vi "SaveAs Document.vi"(8 "error in (no error)":errorcluster, 10 "File Path":path, 11 "Document in":refnum<class "Document.lvclass">) -> (0 "error out":errorcluster, 3 "Document out":refnum<class "Document.lvclass">)   [LabVIEW 2020, in "LabVIEW NPOI.lvlib" / "Document.lvclass"]
doc: "Saves the <b>Document</b> to the given <b>File Path</b>.\n\nNotes:\n - If <b>File Path</b> is empty (default) or is <Not A Path> or is a directory, the VI displays a dialog box from which the user can select a file. Error 43 occurs if you cancel the dialog box. \n - If the <b>File Path</b> already contains a docuement with the same name then that file is overwritten without warning."
uses:
  Document.lvclass
  Document.lvclass/Document.ctl
  Support/Files/Prompt File Dialog.vi
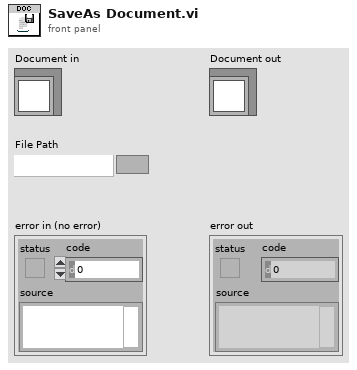
[diagram p1: front panel]
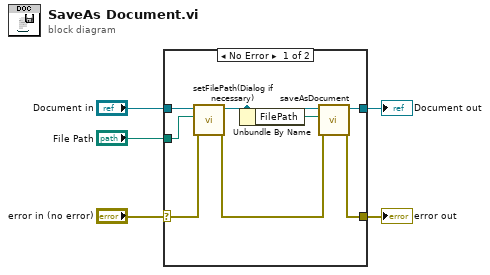
[diagram p0: block diagram]
diagram:
  n1 = case shown="No Error" "error in (no error)" {
    selector: "error in (no error)" -> [w9 w15]
    tunnel: [w12 w15] -> w4
    tunnel: [w13 w14] -> w2
    tunnel: "Document in" -> [w11 w14]
    tunnel: "File Path" -> [w10 _]
    frame No Error {
      n2 = call "setFilePath(Dialog if necessary).vi"("error in (no error)"=w9, "FilePath"=w10, "Document in"=w11) -> ("error out"=w8:errorcluster, "Document out"=w7:refnum<class "Document.lvclass">)  [unwired: 7 in]
      n3 = Unbundle By Name(w7) -> ("FilePath"=w6:path)
      n4 = call-dynamic "saveAsDocument.vi"("error in (no error)"=w8, "File Path"=w6, "Document in"=w7) -> ("error out"=w12:errorcluster, "Document out"=w13:refnum<class "Document.lvclass">)  [unwired: 7 in]
    }
    frame Error {
    }
  }
  "error out" <- w4
  "Document out" <- w2
